vi "Msg Loop.vi"(11 "LVCAM in":refnum<class "LVCAM.lvclass">) -> ()   [LabVIEW 2021, in "LVCAM.lvlib" / "LVCAM.lvclass"]
uses:
  LVCAM.lvclass
  Msg/Msg.lvclass
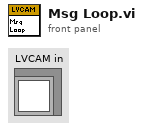
[diagram p1: front panel]
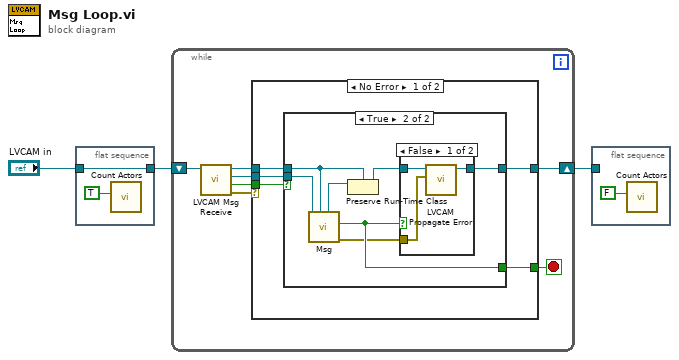
[diagram p0: block diagram]
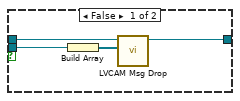
[diagram p2: hidden frame]
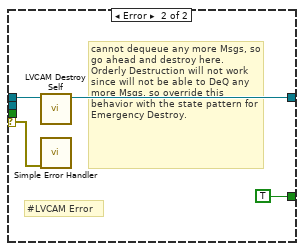
[diagram p4: hidden frame]
diagram:
  n1 = flat-sequence {
    tunnel: [w4] -> w2
    tunnel: "LVCAM in" -> [w4]
    frame #0 {
      n2 = call "Count Actors.vi"("Increment?"=TRUE) -> ()  [unwired: 11 in]
    }
  }
  n3 = while {
    shift-right: [w12] -> w1
    shift-left: w2 -> [w8]
    stop <- w9 stop-if-true
    n4 = call-dynamic "LVCAM Msg Receive.vi"("LVCAM Msg Receive in"=w8) -> ("error out"=w6:errorcluster, "DeQ Msg?"=w10:bool, "Msg"=w11:refnum<class "Msg.lvclass">, "LVCAM Msg Receive out"=w7:refnum<class "LVCAM.lvclass">)  [unwired: 7 in]
    n5 = case shown="No Error" w6 {
      selector: w6 -> [_ w33]
      tunnel: [w13 w35] -> w12
      tunnel: w11 -> [w17 _]
      tunnel: w10 -> [w16 _]
      tunnel: [w15 TRUE ("Destroyed Self?")] -> w9
      tunnel: w7 -> [w14 w36]
      frame No Error {
        n6 = case shown="True" w16 {
          tunnel: w14 -> [w21 w28]
          tunnel: [_ w23] -> w15
          tunnel: [w18 w24] -> w13
          tunnel: w17 -> [w20 w26]
          frame False {
            n7 = Build Array(w20) -> (w19:refnum<class "Msg.lvclass">[])
            n8 = call-dynamic "LVCAM Msg Drop.vi"("Remaining Elements"=w19, "LVCAM Msg Drop in"=w21) -> ("LVCAM Msg Drop out"=w18:refnum<class "LVCAM.lvclass">)  [unwired: 9 in]
          }
          frame True {
            n9 = call-dynamic "Msg.vi"("LVCAM in"=w28, "Msg in"=w26) -> ("error out"=w22:errorcluster, "Destroyed Self?"=w23:bool, "LVCAM out"=w27:refnum<class "LVCAM.lvclass">)  [unwired: 7 in]
            n10 = Preserve Run-Time Class(object in=w27, 2:w28) -> (object out=w25:refnum<class "LVCAM.lvclass">)  [unwired: 1 in, 1 out]
            n11 = case shown="False" w23 {
              tunnel: [w31 w32] -> w24
              tunnel: w25 -> [w30 w32]
              tunnel: w22 -> [w29 _]
              frame False {
                n12 = call-dynamic "LVCAM Propagate Error.vi"("Error"=w29, "LVCAM Propagate Error in"=w30) -> ("LVCAM Propagate Error out"=w31:refnum<class "LVCAM.lvclass">)  [unwired: 8 in, 1 out]
              }
              frame True {
              }
            }
          }
        }
      }
      frame Error {
        # "cannot dequeue any more Msgs, so go ahead and destroy here. Orderly Destruction will not work since will not be able to DeQ any more Msgs, so override this behavior with the state pattern for Emergency Destroy."
        # "#LVCAM Error"
        n13 = call-dynamic "LVCAM Destroy Self.vi"("LVCAM Destroy Self in"=w36) -> ("LVCAM Destroy Self out"=w35:refnum<class "LVCAM.lvclass">)  [unwired: 8 in, 2 out]
        n14 = call <vilib>:"Simple Error Handler.vi"("error in (no error)"=w33) -> ()  [unwired: 4 in, 5 out]
      }
    }
  }
  n15 = flat-sequence {
    tunnel: w1 -> [_]
    frame #0 {
      n16 = call "Count Actors.vi"("Increment?"=FALSE) -> ()  [unwired: 11 in]
    }
  }
